vi "AxisMain.vi"(8 "error in (no error)":errorcluster, 11 "Axis in":refnum<class "Axis.lvclass">) -> (0 "error out":errorcluster, 3 "Axis out":refnum<class "Axis.lvclass">)   [LabVIEW 2020, in "Axis.lvclass"]
uses:
  Axis.lvclass
  AxisMainState.ctl
  C:/Users/Jonathan/Documents/Clearpath SDK/CSharp Examples/CLRWrapper/x64/Debug/CLRWrapper.dll
  CSharp Examples/CLRWrapper/x64/Debug/CLRWrapper.dll
  m_state.ctl
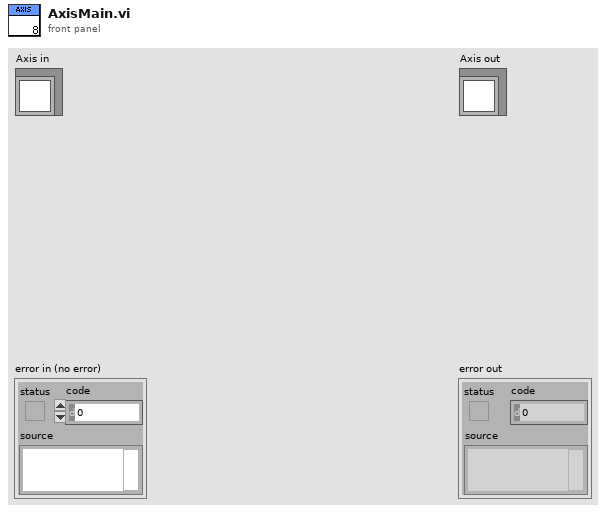
[diagram p1: front panel]
types:
  T1 = typedef "Axis.lvclass/m_state.ctl" = enum16{"STATE_IDLE", "STATE_SEND_MOVE", "STATE_WAIT_FOR_MOVE_DONE", "STATE_EXITED"}
  T2 = typedef "Axis.lvclass/AxisMainState.ctl" = enum16{"Enable", "Home", "AxisStateMachine"}
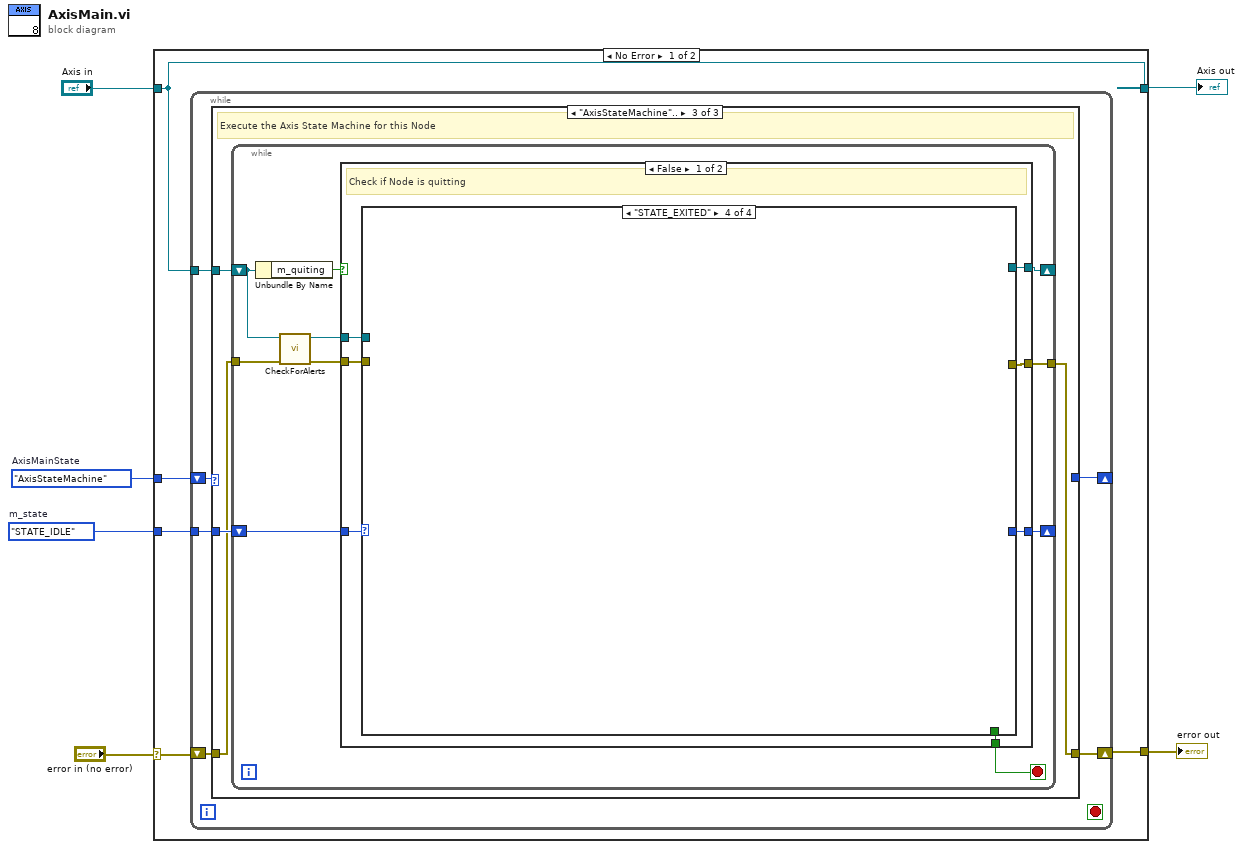
[diagram p0: block diagram]
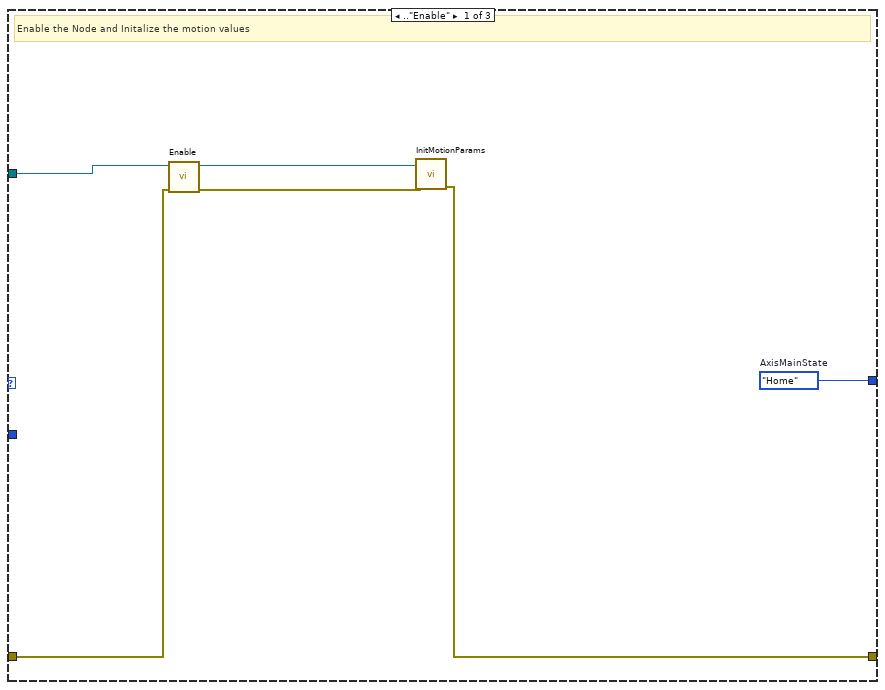
[diagram p2: hidden frame]
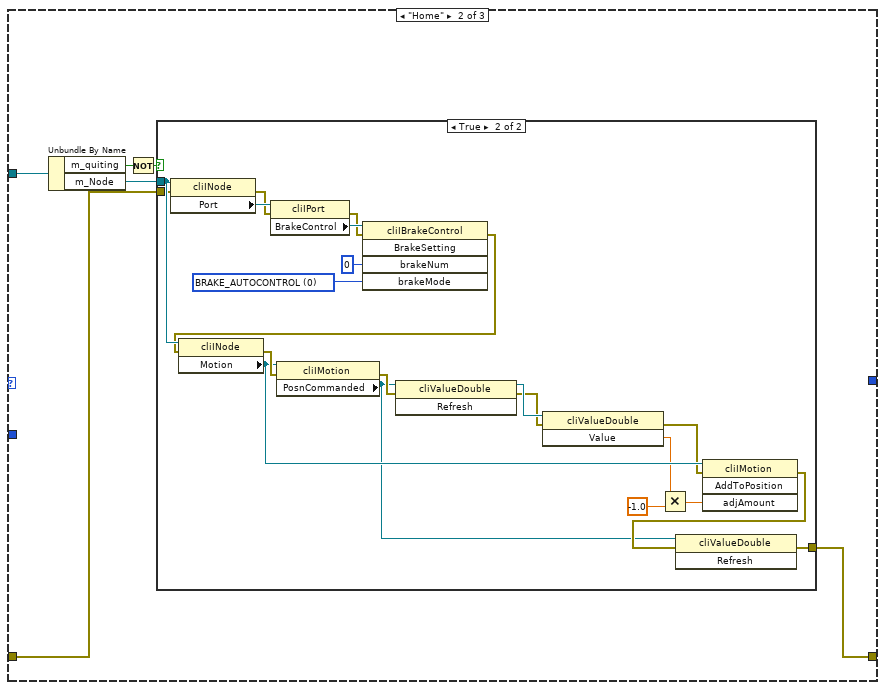
[diagram p3: hidden frame]
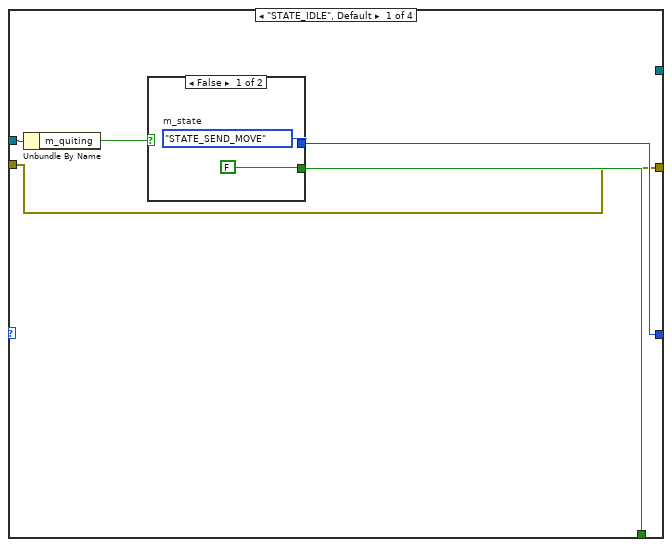
[diagram p5: hidden frame]
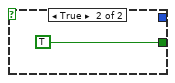
[diagram p6: hidden frame]
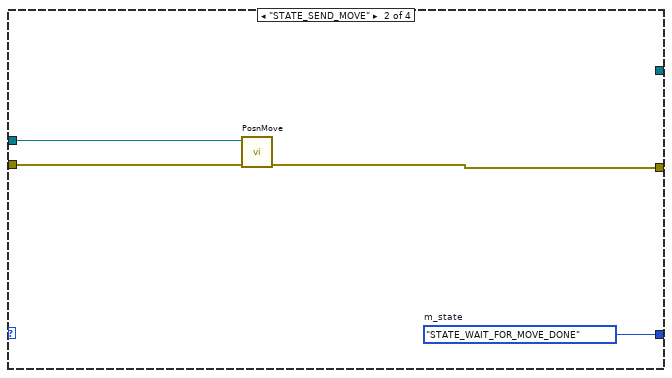
[diagram p7: hidden frame]
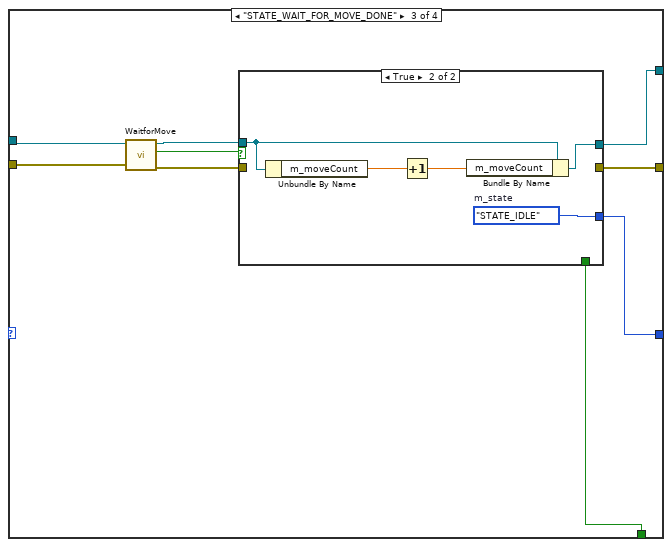
[diagram p8: hidden frame]
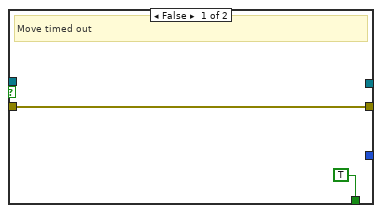
[diagram p9: hidden frame]
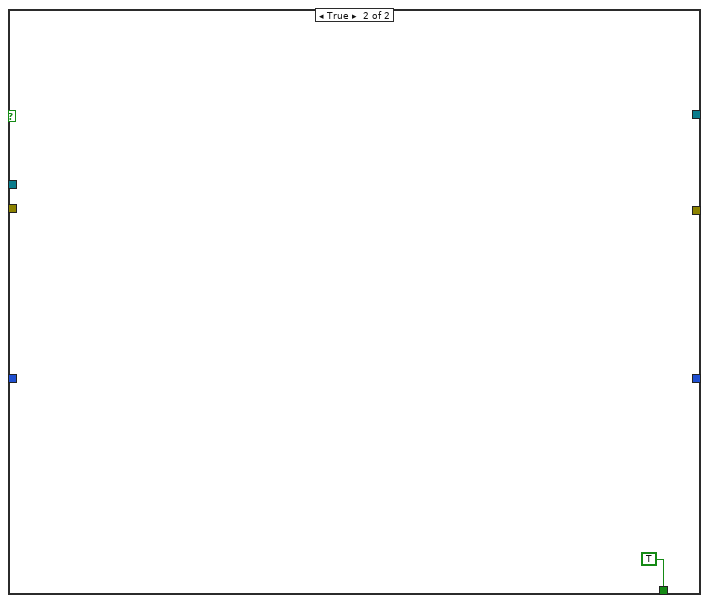
[diagram p10: hidden frame]
diagram:
  w1 = m_state."STATE_IDLE"  # m_state
  w2 = AxisMainState."AxisStateMachine"  # AxisMainState
  n1 = case shown="No Error" "error in (no error)" {
    selector: "error in (no error)" -> [w10 w103]
    tunnel: [w8 w103] -> w5
    tunnel: [w11 w102] -> w3
    tunnel: "Axis in" -> [w11 w102]
    tunnel: w2 -> [w9 _]
    tunnel: w1 -> [w7 _]
    frame No Error {
      n2 = while {
        tunnel: w11 -> [w17]
        shift-right: [w14] -> w8
        shift-left: w10 -> [w16]
        shift-right: [w13] -> _
        shift-left: w9 -> [w15]
        tunnel: w7 -> [w12]
        stop <- _ stop-if-true
        n3 = case shown="\"AxisStateMachine\".." w15 {
          tunnel: w17 -> [w23 w29 w55]
          tunnel: w16 -> [w20 w25 w53]
          tunnel: [w19 w24 w52] -> w14
          tunnel: [w18 _ _] -> w13
          tunnel: w12 -> [_ _ w54]
          frame .."Enable" {
            w18 = AxisMainState."Home"  # AxisMainState
            # "Enable the Node and Initalize the motion values"
            n4 = call "Enable.vi"("error in (no error)"=w20, "Axis in"=w23) -> ("error out"=w21:errorcluster, "Axis out"=w22:refnum<class "Axis.lvclass">)  [unwired: 8 in]
            n5 = call "InitMotionParams.vi"("error in (no error)"=w21, "Axis in"=w22) -> ("error out"=w19:errorcluster)  [unwired: 8 in, 1 out]
          }
          frame "Home" {
            n6 = Unbundle By Name(w29) -> ("m_quiting"=w27:bool, "m_Node"=w26:refnum<k24>)
            n7 = Not(x=w27) -> (.not. x?=w28:bool)
            n8 = case shown="True" w28 {
              tunnel: w26 -> [_ w47]
              tunnel: w25 -> [w30 w41]
              tunnel: [w30 w31] -> w24
              frame False {
              }
              frame True {
                w48 = 0 items=["BRAKE_AUTOCONTROL", "BRAKE_PREVENT_MOTION", "BRAKE_ALLOW_MOTION", "GPO_ON", "GPO_OFF"] ("brakeMode")
                n9 = property class="cliINode"(reference=w47, error in=w41) -> (error out=w44:errorcluster, "Port"=w51:refnum<k24>)  [unwired: 1 out]
                n10 = property class="cliIPort"(reference=w51, error in=w44) -> (error out=w45:errorcluster, "BrakeControl"=w50:refnum<k24>)  [unwired: 1 out]
                n11 = invoke class="cliIBrakeControl" method="BrakeSetting"(reference=w50, error in=w45, "brakeNum"=u64 0, "brakeMode"=w48) -> (error out=w46:errorcluster)  [unwired: 1 in, 4 out]
                n12 = property class="cliINode"(reference=w47, error in=w46) -> (error out=w43:errorcluster, "Motion"=w39:refnum<k24>)  [unwired: 1 out]
                n13 = property class="cliIMotion"(reference=w39, error in=w43) -> (error out=w42:errorcluster, "PosnCommanded"=w32:refnum<k24>)  [unwired: 1 out]
                n14 = invoke class="cliValueDouble" method="Refresh"(reference=w32, error in=w42) -> (reference out=w40:refnum<k24>, error out=w35:errorcluster)  [unwired: 1 in, 1 out]
                n15 = invoke class="cliValueDouble" method="Value"(reference=w40, error in=w35) -> (error out=w34:errorcluster, "Value"=w38:dbl)  [unwired: 1 in, 1 out]
                n16 = Multiply(x=w38, y=-1.0) -> (x*y=w37:dbl)
                n17 = invoke class="cliIMotion" method="AddToPosition"(reference=w39, error in=w34, "adjAmount"=w37) -> (error out=w33:errorcluster)  [unwired: 1 in, 3 out]
                n18 = invoke class="cliValueDouble" method="Refresh"(reference=w32, error in=w33) -> (error out=w31:errorcluster)  [unwired: 1 in, 2 out]
              }
            }
          }
          frame "AxisStateMachine".. {
            # "Execute the Axis State Machine for this Node"
            n19 = while {
              shift-right: [w60] -> _
              shift-left: w54 -> [w63]
              tunnel: w53 -> [w61]
              tunnel: [w57] -> w52
              shift-right: [w56] -> _
              shift-left: w55 -> [w62]
              stop <- w64 stop-if-true
              n20 = Unbundle By Name(w62) -> ("m_quiting"=w65:bool)
              n21 = call "CheckForAlerts.vi"("error in (no error)"=w61, "Axis in"=w62) -> ("error out"=w58:errorcluster, "Axis out"=w59:refnum<class "Axis.lvclass">)  [unwired: 6 in, 2 out]
              n22 = case shown="False" w65 {
                tunnel: [w69 TRUE] -> w64
                tunnel: w63 -> [w72 _]
                tunnel: [w71 _] -> w60
                tunnel: w59 -> [w70 _]
                tunnel: w58 -> [w68 _]
                tunnel: [w67 _] -> w57
                tunnel: [w66 _] -> w56
                frame False {
                  # "Check if Node is quitting"
                  n23 = case shown="\"STATE_EXITED\"" w72 {
                    tunnel: [w75 w81 w88 _] -> w71
                    tunnel: w70 -> [w77 w84 w93 _]
                    tunnel: [w74 _ w85 _] -> w69
                    tunnel: w68 -> [w73 w83 w92 _]
                    tunnel: [w73 w82 w90 _] -> w67
                    tunnel: [_ _ w86 _] -> w66
                    frame "STATE_IDLE", Default {
                      n24 = Unbundle By Name(w77) -> ("m_quiting"=w76:bool)
                      n25 = case shown="False" w76 {
                        tunnel: [w79 _] -> w75
                        tunnel: [FALSE TRUE] -> w74
                        frame False {
                          w79 = m_state."STATE_SEND_MOVE"  # m_state
                        }
                        frame True {
                        }
                      }
                    }
                    frame "STATE_SEND_MOVE" {
                      w81 = m_state."STATE_WAIT_FOR_MOVE_DONE"  # m_state
                      n26 = call "PosnMove.vi"("error in (no error)"=w83, "Axis in"=w84) -> ("error out"=w82:errorcluster)  [unwired: 8 in, 1 out]
                    }
                    frame "STATE_WAIT_FOR_MOVE_DONE" {
                      n27 = call "WaitforMove.vi"("error in (no error)"=w92, "Axis in"=w93) -> ("error out"=w89:errorcluster, "MoveDone"=w91:bool, "Axis out"=w87:refnum<class "Axis.lvclass">)  [unwired: 7 in]
                      n28 = case shown="True" w91 {
                        tunnel: [w95 _] -> w90
                        tunnel: w89 -> [w95 _]
                        tunnel: [_ w100] -> w88
                        tunnel: w87 -> [_ w99]
                        tunnel: [_ w96] -> w86
                        tunnel: [TRUE _] -> w85
                        frame False {
                          # "Move timed out"
                        }
                        frame True {
                          w100 = m_state."STATE_IDLE"  # m_state
                          n29 = Unbundle By Name(w99) -> ("m_moveCount"=w98:dbl)
                          n30 = Increment(x=w98) -> (x+1=w97:dbl)
                          n31 = Bundle By Name(cluster=w99, "m_moveCount"=w97) -> (w96:refnum<class "Axis.lvclass">)
                        }
                      }
                    }
                    frame "STATE_EXITED" {
                    }
                  }
                }
                frame True {
                }
              }
            }
          }
        }
      }
    }
    frame Error {
    }
  }
  "error out" <- w5
  "Axis out" <- w3
